vi "setDAC.vi"(8 "error in (no error)":errorcluster, 10 "DAC Value":u16, 11 "ILCDAC1 in":refnum<class "ILCDAC1.lvclass">) -> (0 "error out":errorcluster, 3 "ILCDAC1 out":refnum<class "ILCDAC1.lvclass">)   [LabVIEW 2015, in "ILCDAC1.lvclass"]
uses:
  ILCDAC1.lvclass
  <userlib>/Common/ILC/ILC/ILC.lvclass
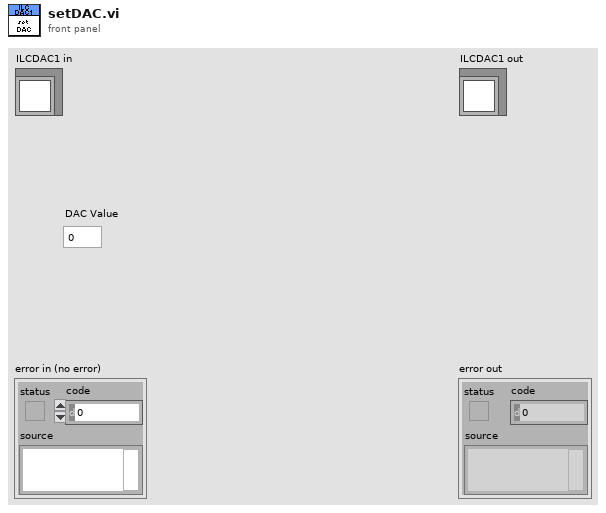
[diagram p1: front panel]
types:
  T1 = typedef "ILCCommon.lvlib/ILCTypedefs.lvlib/OutputData.ctl" = cluster{"Step & Direction":i16, "Blower RPM":u8, "PWM (SSR)":u8, "Ch1":u16, "Ch2":u16, "Ch3":u16, "Ch4":u16}
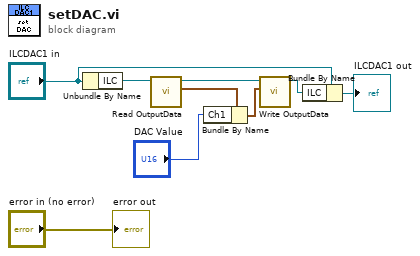
[diagram p0: block diagram]
diagram:
  n1 = Unbundle By Name("ILCDAC1 in") -> ("ILC"=w9:refnum<class "ILC.lvclass">)
  n2 = call <userlib>:"Read OutputData.vi"("ILC in"=w9) -> ("OutputData"=w7:T1, "ILC out"=w8:refnum<class "ILC.lvclass">)  [unwired: 9 in]
  n3 = Bundle By Name(cluster=w7, "Ch1"="DAC Value") -> (w6:T1)
  n4 = call <userlib>:"Write OutputData.vi"("OutputData"=w6, "ILC in"=w8) -> ("ILC out"=w2:refnum<class "ILC.lvclass">)  [unwired: 9 in]
  n5 = Bundle By Name(cluster="ILCDAC1 in", "ILC"=w2) -> (→"ILCDAC1 out":refnum<class "ILCDAC1.lvclass">)
  "error out" <- "error in (no error)"
